vi "Teleop.vi"(10 "Match Info":T4={"Autonomous Elapsed Seconds"=0.0, "TeleOp Elapsed Seconds"=0.0, "Disabled Elapsed Seconds"=0.0, "Visited Autonomous"=FALSE, "Visited TeleOp"=FALSE, "Visited Disabled"=FALSE, "Autonomous Settings"={"Autonomous Style"=enum."Independent", "VI Refnum"=refnum}}, 11 "Call Context":T5) -> ()   [LabVIEW 2016]
doc: "This VI is called for each TeleOp packet received from the DS where the robot is not disabled. It is often used to read from the joysticks and update I/O or to update setpoints for timed control loops. It should complete and return within 20 milliseconds or it may miss DS packets."
uses:
  <vilib>/Rock Robotics/WPI/DriverStation/WPI_DriverStationDerivedRobotMode.ctl
  <vilib>/Rock Robotics/WPI/DriverStation/WPI_DriverStationMatch Info.ctl
  <vilib>/Rock Robotics/WPI/PWM/Servo/WPI_ServoDeviceRef.ctl
  <vilib>/Rock Robotics/SystemInterfaces/DIO/FPGA_DIOPWMChannel.ctl
  <vilib>/Rock Robotics/WPI/PWM/WPI_PWMDeadband.ctl
  <vilib>/Rock Robotics/WPI/Relay/WPI_RelayValue.ctl
  <vilib>/Rock Robotics/WPI/Utilities/WPI_GetSetVariantRefNum.vi
  <vilib>/Rock Robotics/Network Tables/NT Write Boolean Array.vi
  <vilib>/Rock Robotics/Network Tables/NT Write Numeric Array.vi
  <vilib>/Rock Robotics/Network Tables/NT Read Boolean.vi
  <vilib>/Rock Robotics/Network Tables/NT Read Number.vi
  <vilib>/Rock Robotics/WPI/RobotDrive/WPI_RobotDriveArcadeDrive_Standard(NoSaturation).vi
  <vilib>/Rock Robotics/Network Tables/NT Write String.vi
  <vilib>/Rock Robotics/Network Tables/NT Write Boolean.vi
  <vilib>/Rock Robotics/WPI/Power/WPI_Power Get 6Volt Rail Voltage and Current.vi
panel:
  out "Bottom Limit":bool
  out "Top Limit":bool
  out "Y Motor Value":dbl
  out "X Motor Value":dbl
  out "all currents (A)":dbl[](array[numeric])
  out "current (A)":dbl
  out "all currents (A) 2":dbl[](array[numeric])
  out "PDP current (A)":dbl
  out "PDP voltage (V)":dbl
  out "Power (W)":dbl
  out "Energy (J)":dbl
  out "6 volt rail current (A)":dbl
  out "6 volt rail voltage (V)":dbl
  out "5V User Rail Brown Out":bool
  out "6 V User Rail Short":bool
  out "5 V User Rail Short":bool
  out "3.3V User Rail Short":bool
  out "Input Voltage Brown Out":bool
  out "roboRIO input current (A)":dbl
  out "roboRIO input voltage (V)":dbl
  out "Encoder Status":string
  out "Encoder Rate":dbl
  out "Encoder Direction":string
  out "Encoder Distance":dbl
  out "Gripper Position":dbl
  out "Gripper Servo Device Ref":T1={"DeviceStatus"={"status"=FALSE, "code"=0, "source"=""}, "PWM Channel"=enum."Invalid", "DeadBand"={"Name"="", "maxPositivePwm"=0, "minPositivePwm"=0, "centerPwm"=0, "maxNegativePwm"=0, "minNegativePwm"=0, "angularRange"=0}}
  out "Arm Position":dbl
  out "Arm Servo Device Ref":T1={"DeviceStatus"={"status"=FALSE, "code"=0, "source"=""}, "PWM Channel"=enum."Invalid", "DeadBand"={"Name"="", "maxPositivePwm"=0, "minPositivePwm"=0, "centerPwm"=0, "maxNegativePwm"=0, "minNegativePwm"=0, "angularRange"=0}}
  in  "Gripper Scale Factor":dbl=0.004
  in  "Arm Scale Factor":dbl=0.004
  out "Sample Slider 0":dbl(slide) scale=0.0..5.0
  out "Sample Boolean 1":bool
  out "Sample Boolean 0":bool
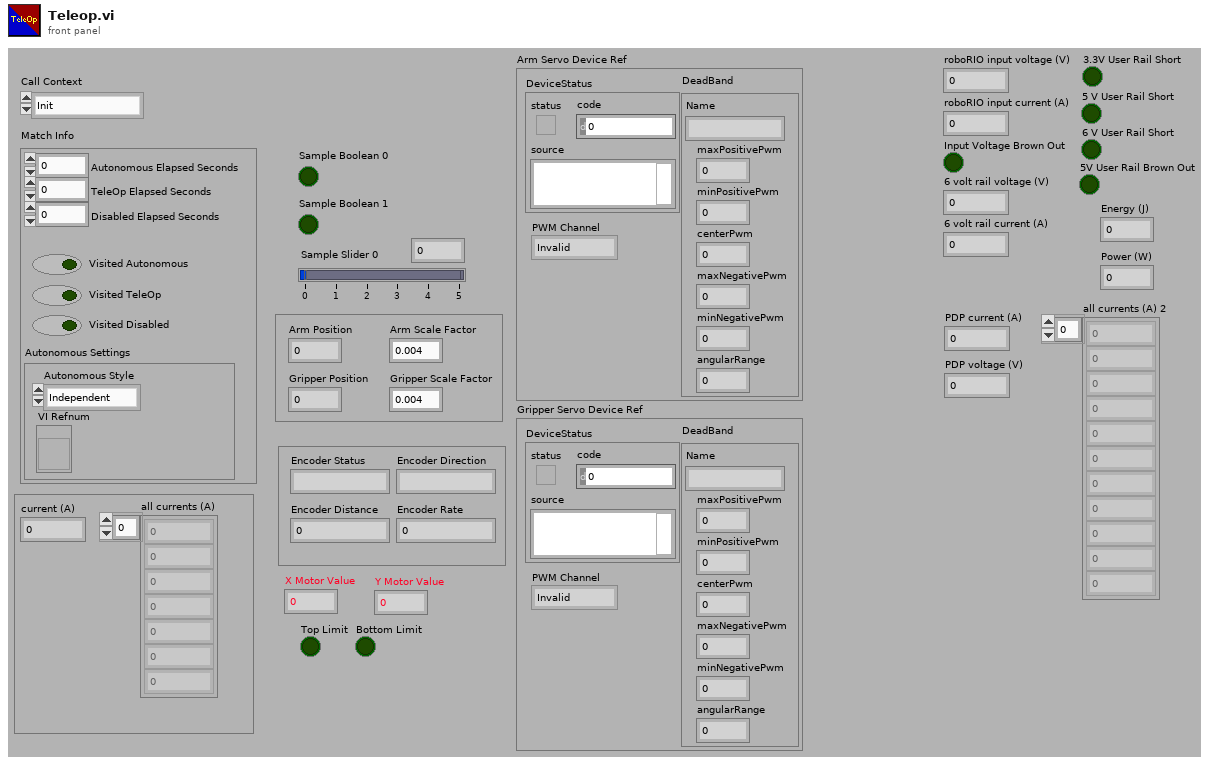
[diagram p1: front panel]
types:
  T1 = typedef "WPI_ServoDeviceRef.ctl" = cluster{"DeviceStatus":errorcluster, "PWM Channel":T2, "DeadBand":T3}
  T2 = typedef "FPGA_DIOPWMChannel.ctl" = enum8{"PWM 0", "PWM 1", "PWM 2", "PWM 3", "PWM 4", "PWM 5", "PWM 6", "PWM 7", "PWM 8", "PWM 9", "PWM MXP 0", "PWM MXP 1", "PWM MXP 2", "PWM MXP 3", "PWM MXP 4", "PWM MXP 5", "PWM MXP 6", "PWM MXP 7", "PWM MXP 8", "PWM MXP 9", "Invalid"}
  T3 = typedef "WPI_PWMDeadband.ctl" = cluster{"Name":string, "maxPositivePwm":i32, "minPositivePwm":i32, "centerPwm":i32, "maxNegativePwm":i32, "minNegativePwm":i32, "angularRange":u16}
  T4 = typedef "WPI_DriverStationMatch Info.ctl" = cluster{"Autonomous Elapsed Seconds":dbl, "TeleOp Elapsed Seconds":dbl, "Disabled Elapsed Seconds":dbl, "Visited Autonomous":bool, "Visited TeleOp":bool, "Visited Disabled":bool, "Autonomous Settings":cluster{"Autonomous Style":enum16{"Iterative", "Independent"}, "VI Refnum":refnum<vi>}}
  T5 = typedef "WPI_DriverStationDerivedRobotMode.ctl" = enum16{"Init", "Execute", "Stop"}
  T6 = typedef "WPI_EncoderDevRef.ctl" = cluster{"DevStatus":errorcluster, "EncoderIndex":T7, "CounterIndex":T8, "DistancePerCount":dbl, "Decoding Type":T9}
  T7 = typedef "FPGA_EncoderIdx.ctl" = enum8{"Enc 0", "Enc 1", "Enc 2", "Enc 3", "Enc 4", "Enc 5", "Enc 6", "Enc 7", "Invalid"}
  T8 = typedef "FPGA_CounterCtrSystemIndex.ctl" = enum8{"Ctr 0", "Ctr 1", "Ctr 2", "Ctr 3", "Ctr 4", "Ctr 5", "Ctr 6", "Ctr 7", "Invalid"}
  T9 = typedef "WPI_EncoderType.ctl" = enum16{"1x", "2x", "4x"}
  T10 = typedef "WPI_RobotDriveDevRef.ctl" = cluster{"DevStatus":errorcluster, "Motors[]":T11[], "Square Inputs":bool, "Max Output":dbl}
  T11 = typedef "WPI_MotorControlDeviceRef.ctl" = cluster{"DeviceStatus":errorcluster, "Type":T12, "PWM":cluster{"PWM Channel":T2, "DeadBand":T3}, "CAN":cluster{"Device Number":u8, "SetOutput VI Ref":variant, "GetOutput VI Ref":variant, "Enable VI Ref":variant, "Disable VI Ref":variant, "Data":variant}, "Invert":bool}
  T12 = typedef "WPI_MotorControlType.ctl" = enum16{"PWM", "CAN"}
  T13 = typedef "WPI_JoystickDevRef.ctl" = cluster{"Device":T14}
  T14 = typedef "WPI_JoystickDeviceEnum.ctl" = enum16{"USB 0", "USB 1", "USB 2", "USB 3", "USB 4", "USB 5"}
  T15 = typedef "WPI_SwitchDevRef.ctl" = cluster{"DevStatus":errorcluster, "DIO Channel":T16, "CntIndex":T8, "Normally Closed":bool}
  T16 = typedef "FPGA_DIOChannel.ctl" = enum8{"DIO 0", "DIO 1", "DIO 2", "DIO 3", "DIO 4", "DIO 5", "DIO 6", "DIO 7", "DIO 8", "DIO 9", "DIO MXP 0", "DIO MXP 1", "DIO MXP 2", "DIO MXP 3", "DIO MXP 4", "DIO MXP 5", "DIO MXP 6", "DIO MXP 7", "DIO MXP 8", "DIO MXP 9", "DIO MXP 10", "DIO MXP 11", "DIO MXP 12", "DIO MXP 13", "DIO MXP 14", "DIO MXP 15", "SPI Port CS1", "SPI Port CS2", "SPI Port CS3", "SPI Port MISO", "SPI Port MOSI", "Invalid"}
  T17 = typedef "WPI_RelayDevRef.ctl" = cluster{"DevStatus":errorcluster, "Relay Channel":T18, "Relay Direction":T19}
  T18 = typedef "FPGA_DIORelayChannel.ctl" = enum8{"Relay 0", "Relay 1", "Relay 2", "Relay 3", "Invalid"}
  T19 = typedef "WPI_RelayDirection.ctl" = enum16{"Both directions", "Forward only", "Reverse only"}
  T20 = typedef "WPI_RelayValue.ctl" = enum16{"Off", "On", "Forward", "Reverse"}
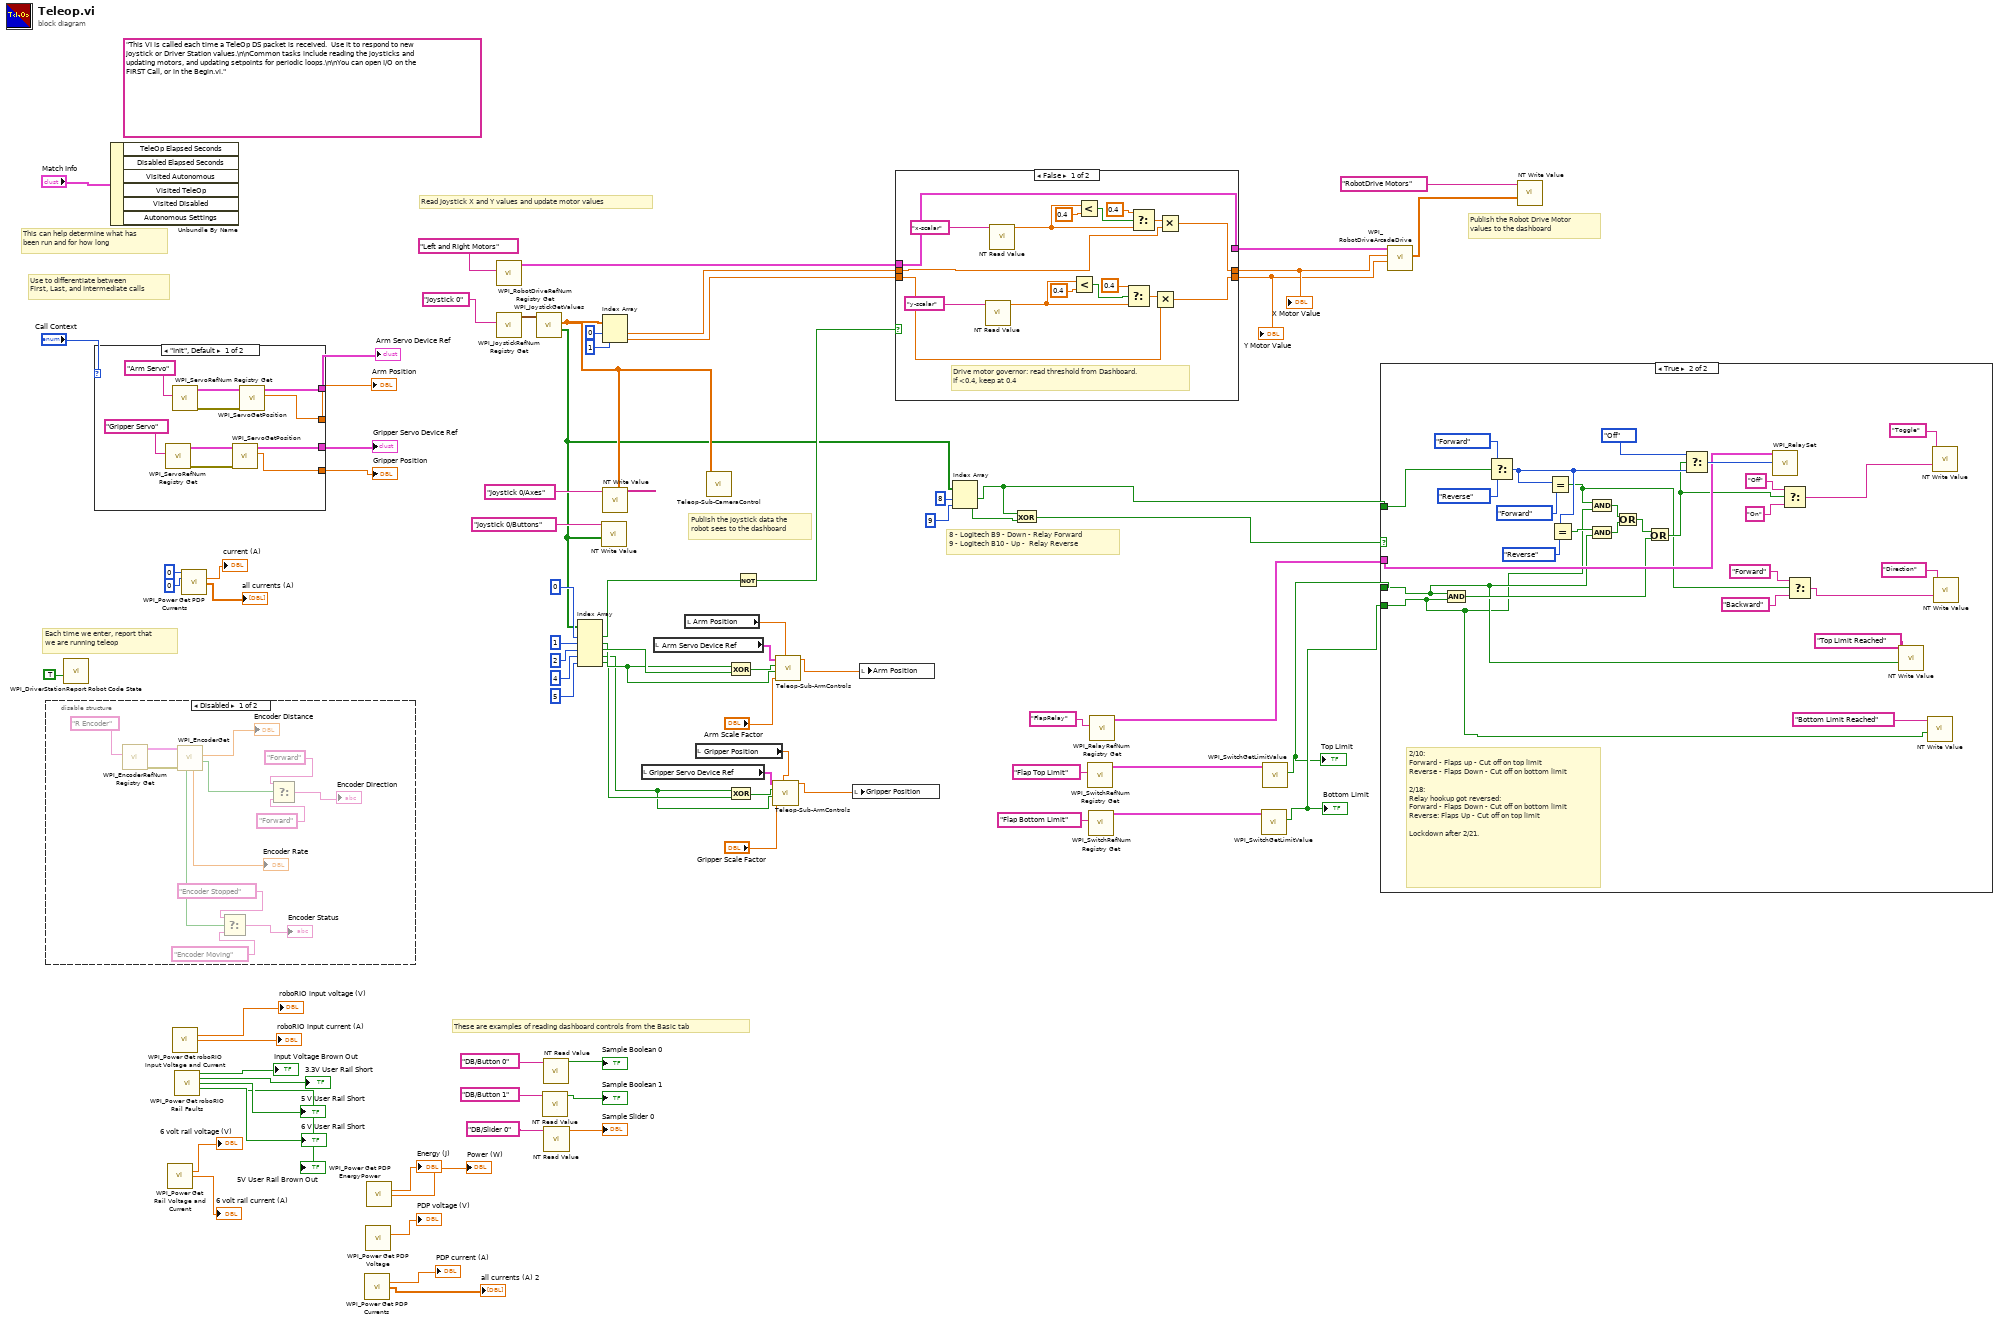
[diagram p0: block diagram]
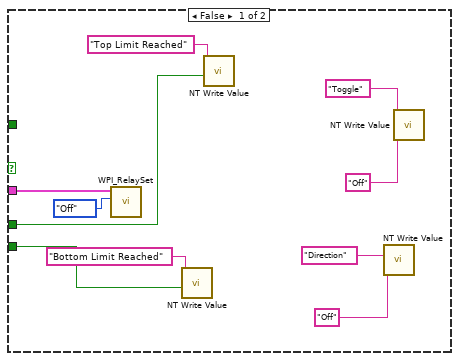
[diagram p2: hidden frame]
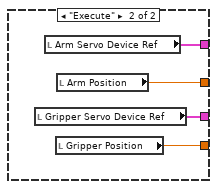
[diagram p4: hidden frame]
diagram:
  (unwired) "This VI is called each time a TeleOp DS packet is received.  Use it to respond to new joystick or Driver Station values.\n\nCommon tasks include reading the joysticks and updating motors, and updating setpoints for periodic loops.\n\nYou can open I/O on the FIRST Call, or in the Begin.vi."
  # "8 - Logitech B9 - Down - Relay Forward\n9 - Logitech B10 - Up -  Relay Reverse"
  # "Publish the Robot Drive Motor\nvalues to the dashboard"
  # "These are examples of reading dashboard controls from the Basic tab"
  # "Publish the joystick data the\nrobot sees to the dashboard"
  # "Each time we enter, report that\nwe are running teleop"
  # "Use to differentiate between\nFirst, Last, and Intermediate calls"
  # "This can help determine what has\nbeen run and for how long"
  # "Read Joystick X and Y values and update motor values"
  n1 = disable-structure shown="Disabled" {
    frame Disabled {
      n2 = call <vilib>:"WPI_EncoderRefNum Registry Get.vi"("refnum name"="R Encoder") -> ("error out"=w94:errorcluster, "EncoderDevRef"=w93:T6)  [unwired: 9 in]
      n3 = call <vilib>:"WPI_EncoderGet.vi"("error in (no error)"=w94, "EncoderDevRef"=w93) -> ("Direction"=w91:bool, "Distance"=→"Encoder Distance":dbl, "Rate"=→"Encoder Rate":dbl, "Stopped"=w85:bool)  [unwired: 4 in, 2 out]
      n4 = Select(t="Encoder Stopped" ("refnum name"), s=w85, f="Encoder Moving" ("refnum name")) -> (s? t:f=→"Encoder Status":string)
      n5 = Select(t="Forward" ("refnum name"), s=w91, f="Forward" ("refnum name")) -> (s? t:f=→"Encoder Direction":string)
    }
    frame Enabled {
    }
  }
  n6 = call <vilib>:"WPI_DriverStationReport Robot Code State.vi"("TeleOp"=TRUE ("Autonomous")) -> ()  [unwired: 10 in, 1 out]
  n7 = case shown="\"Init\", Default" "Call Context" {
    tunnel: [w102 w109] -> w44
    tunnel: [w101 w108] -> w43
    tunnel: [w97 w107] -> w42
    tunnel: [w96 w106] -> w39
    frame "Init", Default {
      n8 = call <vilib>:"WPI_ServoRefNum Registry Get.vi"("refnum name"="Gripper Servo") -> ("error out"=w99:errorcluster, "ServoDeviceRef"=w98:T1)  [unwired: 9 in]
      n9 = call <vilib>:"WPI_ServoRefNum Registry Get.vi"("refnum name"="Arm Servo") -> ("error out"=w104:errorcluster, "ServoDeviceRef"=w105:T1)  [unwired: 9 in]
      n10 = call <vilib>:"WPI_ServoGetPosition.vi"("error in (no error)"=w99, "ServoDeviceRef"=w98) -> ("Position"=w96:dbl, "ServoDeviceRef"=w97:T1)  [unwired: 7 in, 1 out]
      n11 = call <vilib>:"WPI_ServoGetPosition.vi"("error in (no error)"=w104, "ServoDeviceRef"=w105) -> ("Position"=w101:dbl, "ServoDeviceRef"=w102:T1)  [unwired: 7 in, 1 out]
    }
    frame "Execute" {
      n12 = local read "Gripper Servo Device Ref"() -> (w107:T1)
      n13 = local read "Arm Servo Device Ref"() -> (w109:T1)
      n14 = local read "Gripper Position"() -> (w106:dbl)
      n15 = local read "Arm Position"() -> (w108:dbl)
    }
  }
  "Arm Servo Device Ref" <- w44
  "Arm Position" <- w43
  "Gripper Servo Device Ref" <- w42
  "Gripper Position" <- w39
  n16 = Unbundle By Name("Match Info") -> ()  [unwired: 6 out]
  n17 = call-poly <vilib>:"WPI_Power Get Rail Voltage and Current.vi"() -> ("6 volt rail voltage (V)"=→"6 volt rail voltage (V)":dbl, "6 volt rail current (A)"=→"6 volt rail current (A)":dbl)  [unwired: 13 in, 1 out]
  n18 = call <vilib>:"WPI_Power Get roboRIO Input Voltage and Current.vi"() -> ("roboRIO input voltage (V)"=→"roboRIO input voltage (V)":dbl, "roboRIO input current (A)"=→"roboRIO input current (A)":dbl)  [unwired: 13 in, 1 out]
  n19 = call <vilib>:"WPI_Power Get roboRIO Rail Faults.vi"() -> ("Input Voltage Brown Out"=→"Input Voltage Brown Out":bool, "3.3V User Rail Short"=→"3.3V User Rail Short":bool, "5 V User Rail Short"=→"5 V User Rail Short":bool, "6 V User Rail Short"=→"6 V User Rail Short":bool, "5V User Rail Brown Out"=→"5V User Rail Brown Out":bool)  [unwired: 10 in, 1 out]
  n20 = call <vilib>:"WPI_Power Get PDP Currents.vi"("Power Distribution Panel (0)"=u8 0, "PDP Channel"=0) -> ("current (A)"=→"current (A)":dbl, "all currents (A)"=→"all currents (A)":dbl[])  [unwired: 11 in, 1 out]
  n21 = call <vilib>:"WPI_Power Get PDP Currents.vi"() -> ("current (A)"=→"PDP current (A)":dbl, "all currents (A)"=→"all currents (A) 2":dbl[])  [unwired: 13 in, 1 out]
  n22 = call <vilib>:"WPI_Power Get PDP Voltage.vi"() -> ("voltage (V)"=→"PDP voltage (V)":dbl)  [unwired: 14 in, 1 out]
  n23 = call <vilib>:"WPI_Power Get PDP EnergyPower.vi"() -> ("Energy (J)"=→"Energy (J)":dbl, "Power (W)"=→"Power (W)":dbl)  [unwired: 13 in, 1 out]
  n24 = call <vilib>:"WPI_RobotDriveRefNum Registry Get.vi"("refnum name"="Left and Right Motors") -> ("RobotDriveDevRef"=w80:T10)  [unwired: 1 in, 9 out]
  n25 = call <vilib>:"WPI_JoystickRefNum Registry Get.vi"("refnum name"="Joystick 0") -> ("JoystickDevRef"=w77:T13)  [unwired: 1 in, 9 out]
  n26 = call <vilib>:"WPI_JoystickGetValues.vi"("JoystickDevRef"=w77) -> ("Buttons"=w14:bool[], "Axes"=w66:dbl[])  [unwired: 6 in, 3 out]
  n27 = call-poly <vilib>:"NT Read Value.vi"("Name"="DB/Button 1" ("refnum name")) -> ("Boolean"=→"Sample Boolean 1":bool)  [unwired: 9 in, 1 out]
  n28 = call-poly <vilib>:"NT Read Value.vi"("Name"="DB/Button 0" ("refnum name")) -> ("Boolean"=→"Sample Boolean 0":bool)  [unwired: 9 in, 1 out]
  n29 = call-poly <vilib>:"NT Read Value.vi"("Name"="DB/Slider 0" ("refnum name")) -> ("Numeric"=→"Sample Slider 0":dbl)  [unwired: 9 in, 1 out]
  n30 = Index Array(array=w14, index #1=0 ("index"), index #2=1 ("index"), index #3=2 ("index"), index #4=4 ("index"), index #5=5 ("index")) -> (element #1=w59:bool, element #2=w51:bool, element #3=w53:bool, element #4=w46:bool, element #5=w47:bool)
  n31 = call-poly <vilib>:"NT Write Value.vi"("Boolean Array"=w14, "Name"="Joystick 0/Buttons") -> ()  [unwired: 9 in, 1 out]
  n32 = Index Array(array=w66, index #1=0 ("index"), index #2=1 ("index")) -> (element #1=w79:dbl, element #2=w75:dbl)
  n33 = call-poly <vilib>:"NT Write Value.vi"("Numeric Array"=w66, "Name"="Joystick 0/Axes") -> ()  [unwired: 9 in, 1 out]
  n34 = local read "Gripper Servo Device Ref"() -> (w37:T1)
  n35 = local read "Arm Servo Device Ref"() -> (w38:T1)
  n36 = local read "Arm Position"() -> (w36:dbl)
  n37 = local read "Gripper Position"() -> (w35:dbl)
  n38 = call "Teleop-Sub-CameraControl.vi"("Axes"=w66) -> ()  [unwired: 11 in]
  n39 = Exclusive Or(1:w53, 2:w51) -> (0:w52:bool)
  n40 = Exclusive Or(1:w47, 2:w46) -> (0:w48:bool)
  n41 = Not(x=w59) -> (.not. x?=w58:bool)
  n42 = call "Teleop-Sub-ArmControls.vi"("ServoDeviceRef"=w37, "Move Arm?"=w48, "Go Up?"=w46, "Scale Factor"="Gripper Scale Factor", "Position In"=w35) -> ("Position"=w40:dbl)  [unwired: 5 in]
  n43 = call "Teleop-Sub-ArmControls.vi"("ServoDeviceRef"=w38, "Move Arm?"=w52, "Go Up?"=w51, "Scale Factor"="Arm Scale Factor", "Position In"=w36) -> ("Position"=w41:dbl)  [unwired: 5 in]
  n44 = local write "Gripper Position"(w40) -> ()
  n45 = local write "Arm Position"(w41) -> ()
  n46 = case shown="False" w58 {
    tunnel: w80 -> [w126 w129]
    tunnel: w79 -> [w125 w128]
    tunnel: w75 -> [w124 w127]
    tunnel: [w126 w129] -> w63
    tunnel: [w122 w128] -> w62
    tunnel: [w123 w127] -> w61
    frame False {
      # "Drive motor governor: read threshold from Dashboard. \nIf <0.4, keep at 0.4"
      n47 = call-poly <vilib>:"NT Read Value.vi"("Name"="y-scalar") -> ("Numeric"=w111:dbl)  [unwired: 9 in, 1 out]
      n48 = call-poly <vilib>:"NT Read Value.vi"("Name"="x-scalar") -> ("Numeric"=w116:dbl)  [unwired: 9 in, 1 out]
      n49 = Less?(x=w111, y=0.4) -> (x < y?=w113:bool)
      n50 = Less?(x=w116, y=0.4) -> (x < y?=w118:bool)
      n51 = Select(t=0.4 ("y"), s=w113, f=w111) -> (s? t:f=w110:dbl)
      n52 = Select(t=0.4, s=w118, f=w116) -> (s? t:f=w115:dbl)
      n53 = Multiply(x=w110, y=w124) -> (x*y=w123:dbl)
      n54 = Multiply(x=w115, y=w125) -> (x*y=w122:dbl)
    }
    frame True {
      # "If button is not pressed, pass Axes positions \nthrough."
    }
  }
  "X Motor Value" <- w62
  "Y Motor Value" <- w61
  n55 = Index Array(array=w14, index #1=8 ("index"), index #2=9 ("index")) -> (element #1=w9:bool, element #2=w11:bool)
  n56 = Exclusive Or(1:w11, 2:w9) -> (0:w10:bool)
  n57 = call <vilib>:"WPI_SwitchRefNum Registry Get.vi"("refnum name"="Flap Top Limit") -> ("SwitchDevRef"=w4:T15)  [unwired: 9 in, 1 out]
  n58 = call <vilib>:"WPI_SwitchRefNum Registry Get.vi"("refnum name"="Flap Bottom Limit") -> ("SwitchDevRef"=w3:T15)  [unwired: 9 in, 1 out]
  n59 = call <vilib>:"WPI_RelayRefNum Registry Get.vi"("refnum name"="FlapRelay") -> ("RelayDevRef"=w7:T17)  [unwired: 9 in, 1 out]
  n60 = call <vilib>:"WPI_SwitchGetLimitValue.vi"("SwitchDevRef"=w3) -> ("Switch Pressed"=w2:bool)  [unwired: 8 in, 2 out]
  "Bottom Limit" <- w2
  n61 = call <vilib>:"WPI_SwitchGetLimitValue.vi"("SwitchDevRef"=w4) -> ("Switch Pressed"=w1:bool)  [unwired: 8 in, 2 out]
  "Top Limit" <- w1
  n62 = case shown="True" w10 {
    tunnel: w9 -> [_ w165]
    tunnel: w7 -> [w139 w153]
    tunnel: w1 -> [w131 w141]
    tunnel: w2 -> [w130 w140]
    frame False {
      n63 = call <vilib>:"WPI_RelaySet.vi"("RelayValue"=WPI_RelayValue."Off", "RelayDevRef"=w139) -> ()  [unwired: 8 in, 2 out]
      n64 = call-poly <vilib>:"NT Write Value.vi"("Boolean"=w130, "Name"="Bottom Limit Reached") -> ()  [unwired: 9 in, 1 out]
      n65 = call-poly <vilib>:"NT Write Value.vi"("Boolean"=w131, "Name"="Top Limit Reached") -> ()  [unwired: 9 in, 1 out]
      n66 = call-poly <vilib>:"NT Write Value.vi"("String"="Off", "Name"="Direction") -> ()  [unwired: 9 in, 1 out]
      n67 = call-poly <vilib>:"NT Write Value.vi"("String"="Off", "Name"="Toggle") -> ()  [unwired: 9 in, 1 out]
    }
    frame True {
      # "2/10: \nForward - Flaps up - Cut off on top limit\nReverse - Flaps Down - Cut off on bottom limit\n\n2/18:\nRelay hookup got reversed:\nForward - Flaps Down - Cut off on bottom limit\nReverse: Flaps Up - Cut off on top limit\n\nLockdown after 2/21."
      n68 = And(x=w141, y=w140) -> (x .and. y?=w142:bool)
      n69 = Select(t=WPI_RelayValue."Forward" ("RelayValue"), s=w165, f=WPI_RelayValue."Reverse" ("RelayValue")) -> (s? t:f=w159:T20)
      n70 = Equal?(x=w159, y=WPI_RelayValue."Forward" ("RelayValue")) -> (x = y?=w146:bool)
      n71 = Equal?(x=w159, y=WPI_RelayValue."Reverse" ("RelayValue")) -> (x = y?=w158:bool)
      n72 = And(x=w146, y=w140) -> (x .and. y?=w157:bool)
      n73 = And(x=w158, y=w141) -> (x .and. y?=w156:bool)
      n74 = Or(x=w157, y=w156) -> (x .or. y?=w155:bool)
      n75 = Or(x=w155, y=w142) -> (x .or. y?=w152:bool)
      n76 = Select(t=WPI_RelayValue."Off" ("RelayValue"), s=w152, f=w159) -> (s? t:f=w154:T20)
      n77 = call <vilib>:"WPI_RelaySet.vi"("RelayValue"=w154, "RelayDevRef"=w153) -> ()  [unwired: 8 in, 2 out]
      n78 = Select(t="Off" ("String"), s=w152, f="On" ("String")) -> (s? t:f=w149:string)
      n79 = Select(t="Forward" ("String"), s=w146, f="Backward" ("String")) -> (s? t:f=w145:string)
      n80 = call-poly <vilib>:"NT Write Value.vi"("Boolean"=w141, "Name"="Top Limit Reached") -> ()  [unwired: 9 in, 1 out]
      n81 = call-poly <vilib>:"NT Write Value.vi"("Boolean"=w140, "Name"="Bottom Limit Reached") -> ()  [unwired: 9 in, 1 out]
      n82 = call-poly <vilib>:"NT Write Value.vi"("String"=w149, "Name"="Toggle") -> ()  [unwired: 9 in, 1 out]
      n83 = call-poly <vilib>:"NT Write Value.vi"("String"=w145, "Name"="Direction") -> ()  [unwired: 9 in, 1 out]
    }
  }
  n84 = call-poly <vilib>:"WPI_RobotDriveArcadeDrive.vi"("Y axis value"=w61, "X axis value"=w62, "RobotDriveDevRef"=w63) -> ("Motor Values"=w64:dbl[])  [unwired: 6 in, 2 out]
  n85 = call-poly <vilib>:"NT Write Value.vi"("Numeric Array"=w64, "Name"="RobotDrive Motors") -> ()  [unwired: 9 in, 1 out]
